vi "VLC - Fullscreen.vi"() -> ()   [LabVIEW 2016]
uses:
  System.Windows.Forms
panel:
  in  "PictureBox":refnum<k24>(container)
  # "!!!UPDATE CAMERA NAME and AUDIO Input to match your SYSTEM!!!"
  # "http://www.videolan.org/doc/vlc-user-guide/en/ch04.html\nhttp://www.videolan.org/developers/vlc/doc/doxygen/html/group__libvlc__video.html#ga26892692dcb079743c9c7e0df3308ea4"
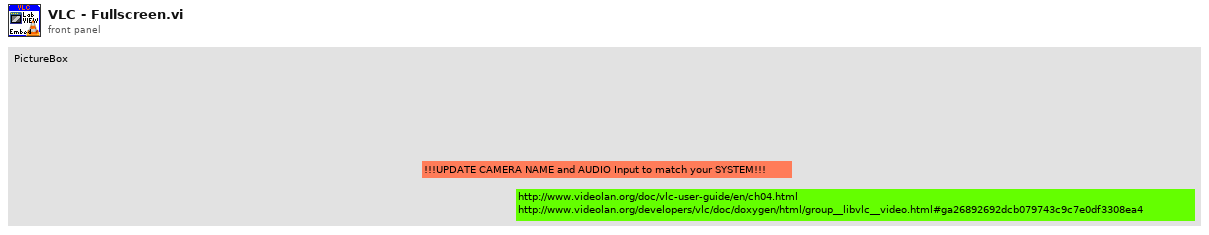
[diagram p1: front panel]
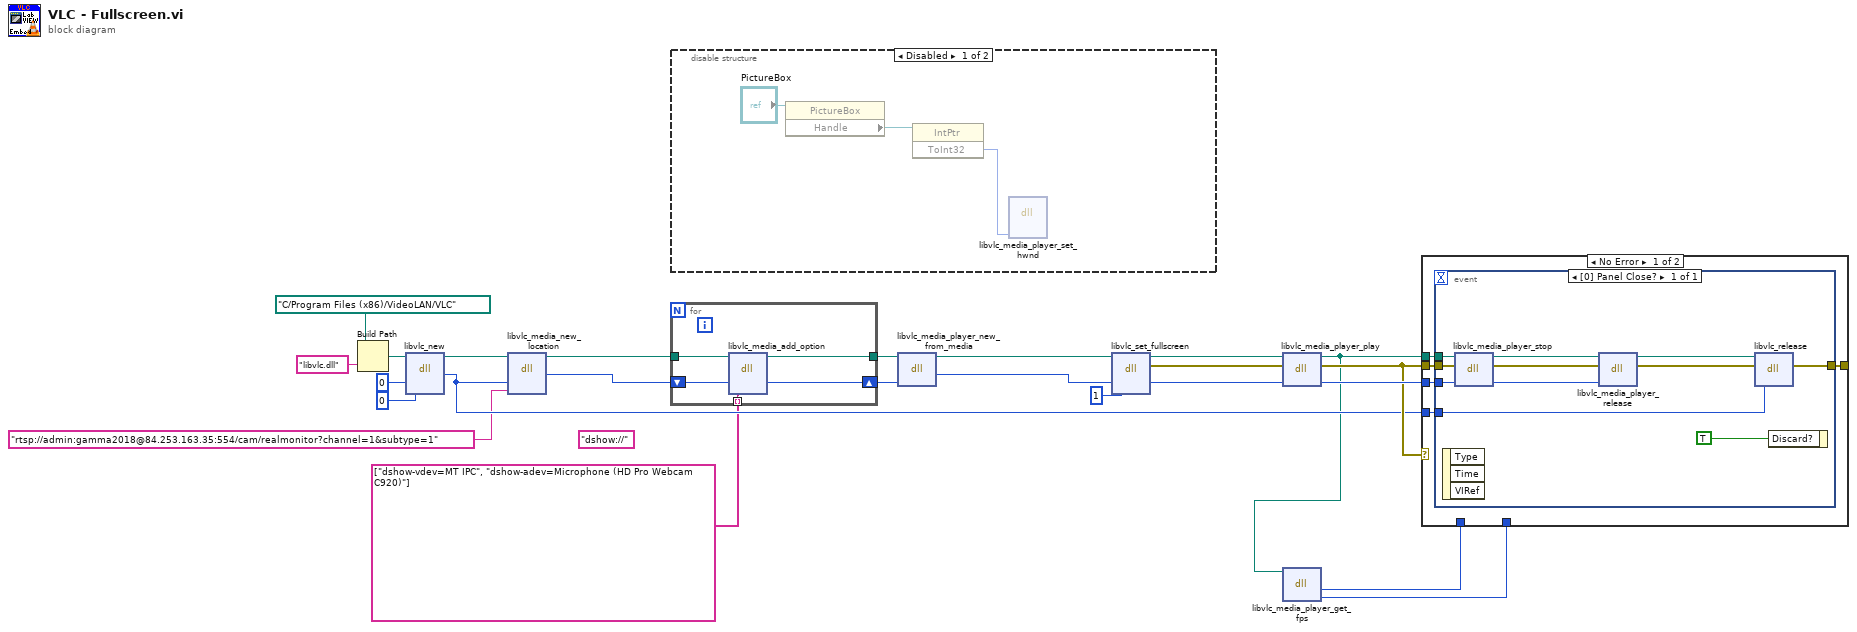
[diagram p0: block diagram]
diagram:
  (unwired) "dshow://" ("Media Source")
  n1 = Build Path(base path=path "C:/Program Files (x86)/VideoLAN/VLC", name or relative path="libvlc.dll") -> (appended path=w17:path)
  n2 = dll-call lib="C:/Program Files (x86)/VideoLAN/VLC/libvlc.dll" fn="libvlc_new"(path in=w17, "argc"=i16 0, "argv"=u8 0) -> (path out=w15:path, "return type"=w14:i32)  [unwired: 4 in, 1 out]
  n3 = dll-call lib="C:/Program Files (x86)/VideoLAN/VLC/libvlc.dll" fn="libvlc_media_new_location"(path in=w15, "p_instance"=w14, "path"="rtsp://admin:gamma2018@84.253.163.35:554/cam/realmonitor?channel=1&subtype=1" ("Media Source")) -> (path out=w11:path, "return type"=w10:i32)  [unwired: 4 in, 1 out]
  n4 = for {
    tunnel: w11 -> [w29]
    tunnel: [w27] -> w9
    shift-right: [w26] -> w8
    shift-left: w10 -> [w28]
    tunnel: string[] ["dshow-vdev=MT IPC", "dshow-adev=Microphone (HD Pro Webcam C920)"] -> [w25] mode=indexing
    n5 = dll-call lib="C:/Program Files (x86)/VideoLAN/VLC/libvlc.dll" fn="libvlc_media_add_option"(path in=w29, "p_md"=w28, "ppsz_options"=w25) -> (path out=w27:path, "p_md"=w26:i32)  [unwired: 4 in, 1 out]
  }
  n6 = disable-structure shown="Disabled" {
    frame Disabled {
      n7 = property class="PictureBox"(reference="PictureBox") -> ("Handle"=w31:refnum<k24>)  [unwired: 1 in, 2 out]
      n8 = invoke class="IntPtr" method="ToInt32"(reference=w31) -> ("ToInt32"=w30:i32)  [unwired: 2 in, 2 out]
      n9 = dll-call lib="C:/Program Files (x86)/VideoLAN/VLC/libvlc.dll" fn="libvlc_media_player_set_hwnd"("drawable"=w30) -> ()  [unwired: 7 in, 2 out]
    }
    frame Enabled {
    }
  }
  n10 = dll-call lib="C:/Program Files (x86)/VideoLAN/VLC/libvlc.dll" fn="libvlc_media_player_new_from_media"(path in=w9, "p_md"=w8) -> (path out=w4:path, "return type"=w7:i32)  [unwired: 3 in, 1 out]
  n11 = dll-call lib="C:/Program Files (x86)/VideoLAN/VLC/libvlc.dll" fn="libvlc_set_fullscreen"(path in=w4, "p_mi"=w7, "fullscreen"=1) -> (path out=w19:path, error out=w23:errorcluster, "p_mi"=w22:i32)  [unwired: 4 in]
  n12 = dll-call lib="C:/Program Files (x86)/VideoLAN/VLC/libvlc.dll" fn="libvlc_media_player_play"(path in=w19, error in=w23, "p_mi"=w22) -> (path out=w3:path, error out=w16:errorcluster, "p_mi"=w24:i32)  [unwired: 2 in]
  n13 = dll-call lib="C:/Program Files (x86)/VideoLAN/VLC/libvlc.dll" fn="libvlc_media_player_get_fps"(path in=w3) -> ("return type"=w2:i32, "p_mi"=w1:i32)  [unwired: 3 in, 2 out]
  n14 = case shown="No Error" w16 {
    tunnel: w14 -> [w37 _]
    tunnel: w24 -> [w36 _]
    tunnel: w16 -> [w35 w49]
    tunnel: w3 -> [w34 _]
    tunnel: [w33 w49] -> _
    tunnel: w2 -> [_ _]
    tunnel: w1 -> [_ _]
    frame No Error {
      n15 = event shown="[0] Panel Close?" {
        selector: _ -> [_]
        dyn-events: _ -> [_]
        timeout: _ -> [_]
        tunnel: w35 -> [w48]
        tunnel: w36 -> [w47]
        tunnel: w37 -> [w43]
        tunnel: w34 -> [w41]
        tunnel: [w38] -> w33
        event Panel Close? {
          n16 = event-data() -> ()  [unwired: 1 in, 3 out]
          n17 = dll-call lib="C:/Program Files (x86)/VideoLAN/VLC/libvlc.dll" fn="libvlc_media_player_stop"(path in=w41, error in=w48, "p_mi"=w47) -> (path out=w40:path, error out=w46:errorcluster, "p_mi"=w45:i32)  [unwired: 2 in]
          n18 = dll-call lib="C:/Program Files (x86)/VideoLAN/VLC/libvlc.dll" fn="libvlc_media_player_release"(path in=w40, error in=w46, "p_mi"=w45) -> (path out=w39:path, error out=w44:errorcluster)  [unwired: 3 in]
          n19 = dll-call lib="C:/Program Files (x86)/VideoLAN/VLC/libvlc.dll" fn="libvlc_release"(path in=w39, error in=w44, "p_instnace"=w43) -> (error out=w38:errorcluster)  [unwired: 3 in, 1 out]
          n20 = event-data("Discard?"=TRUE) -> ()  [unwired: 1 in, 1 out]
        }
      }
    }
    frame Error {
    }
  }
